vi "ziGetVoltageCalc.vi"   [LabVIEW 2018, in "Zurich Instruments LabOne.lvlib"]
uses:
  Zurich Instruments LabOne.lvlib
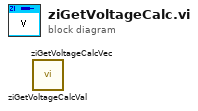
[diagram p0: block diagram]
diagram:
  n1 = call "ziGetVoltageCalcVal.vi"() -> ()  [unwired: 11 in, 1 out]
  n2 = call "ziGetVoltageCalcVec.vi"() -> ()  [unwired: 11 in, 1 out]
